vi "Get Status Color.vi"(1 "Status":T1=enum."Error") -> (0 "Color":u32(colorbox))   [LabVIEW 2015, in "Execution.lvclass"]
uses:
  Execution.lvclass
  Step/STEP_STATUS.ctl
  Step.lvclass
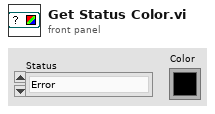
[diagram p1: front panel]
types:
  T1 = typedef "Step.lvclass/STEP_STATUS.ctl" = enum16{"Skipped", "Done", "Passed", "Failed", "Error"}
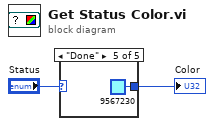
[diagram p0: block diagram]
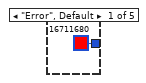
[diagram p2: hidden frame]
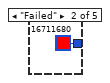
[diagram p3: hidden frame]
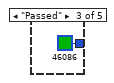
[diagram p4: hidden frame]
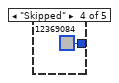
[diagram p5: hidden frame]
diagram:
  n1 = case shown="\"Done\"" "Status" {
    tunnel: [u32 16711680 ("Color") u32 16711680 ("Color") u32 46086 ("Color") u32 12369084 ("Color") u32 9567230 ("Color")] -> w1
    frame "Error", Default {
    }
    frame "Failed" {
    }
    frame "Passed" {
    }
    frame "Skipped" {
    }
    frame "Done" {
    }
  }
  "Color" <- w1
